vi "RW_Redis.vi"(8 "error in":errorcluster, 10 "command":string="PING", 11 "refnum":refnum<vi>) -> (0 "error out":errorcluster, 2 "Data":T1)   [LabVIEW 2020]
uses:
  Controls/redis-data.ctl
panel:
  in  "refnum":cluster{"host":string, "port":u16}={"host"="localhost", "port"=6379}
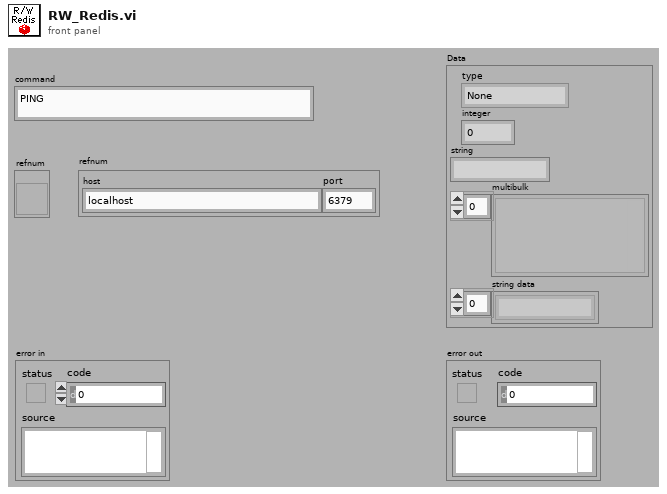
[diagram p1: front panel]
types:
  T1 = typedef "redis-data.ctl" = cluster{"type":enum16{"None", "Error", "Status", "Nil", "Integer", "String", "Multibulk"}, "integer":i64, "string":string, "multibulk":variant[], "string data":string[]}
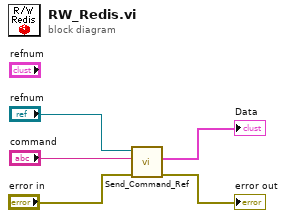
[diagram p0: block diagram]
diagram:
  n1 = call "Send_Command_Ref.vi"("error in"="error in", "command"="command", "refnum in"="refnum") -> ("error out"=→"error out":errorcluster, "Data"=→"Data":T1)  [unwired: 7 in]
